vi "bloc_decodage.vi"(10 "sigma2":string, 11 "Array":cdb[](array[numeric])) -> (1 "sortie complexe":string, 2 "sortie décodeur":string, 3 "output bit stream":i8[](array[numeric]))   [LabVIEW 2018]
uses:
  <vilib>/addons/Modulation/niDMT.lvlib
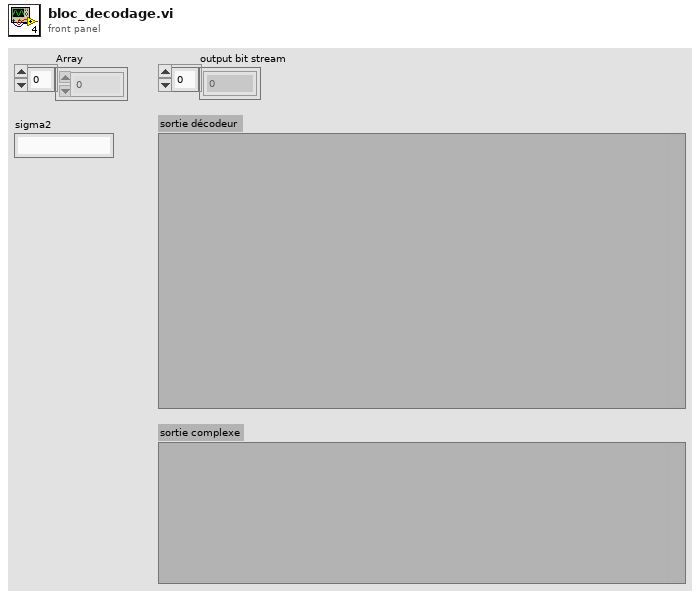
[diagram p1: front panel]
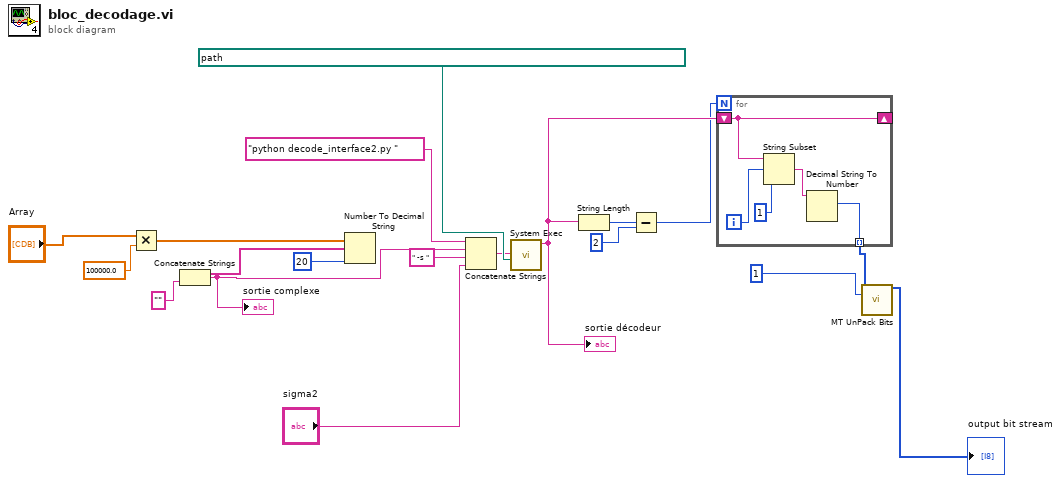
[diagram p0: block diagram]
diagram:
  n1 = Multiply(x="Array", y=100000.0 ("x")) -> (x*y=w5:cdb[])
  n2 = Number To Decimal String(number=w5, width (-)=i16 20) -> (decimal integer string=w1:string[])
  n3 = Concatenate Strings(w1, "") -> (w7:string)
  "sortie complexe" <- w7
  n4 = Concatenate Strings("python decode_interface2.py ", w7, " -s " ("string"), "sigma2") -> (w8:string)
  n5 = call <vilib>:"System Exec.vi"("working directory"=path "C:/Users/pc-labview/Desktop/Levi/Turbo-Codes/Implémentation perso Python/BCJR_OO", "command line"=w8) -> ("standard output"=w17:string)  [unwired: 4 in, 5 out]
  "sortie décodeur" <- w17
  n6 = String Length(string=w17) -> (length=w14:i32)
  n7 = Subtract(x=w14, y=2) -> (x-y=w16:i32)
  n8 = for {
    N: w16 -> [_]
    tunnel: [w21] -> w13 mode=indexing
    shift-right: [w20] -> _
    shift-left: w17 -> [w20]
    i -> [w24]
    n9 = String Subset(string=w20, offset (0)=w24, length (rest)=1) -> (substring=w22:string)
    n10 = Decimal String To Number(string=w22) -> (number=w21:i32)  [unwired: 2 in, 1 out]
  }
  n11 = call <vilib>:"MT UnPack Bits.vi"("input integers"=w13, "bits per integer"=1) -> ("output bit stream"=→"output bit stream":i8[])  [unwired: 12 in, 1 out]
